vi "-Build_Query_Error.vi"(8 "error in (no error)":errorcluster, 11 "Postgres Connector In":refnum<class "Postgres Connector.lvclass">) -> (0 "error out":errorcluster, 3 "Postgres Connector Out":refnum<class "Postgres Connector.lvclass">)   [LabVIEW 2020, in "Postgres Connector.lvclass"]
doc: "This VI return the error associated with a query"
uses:
  Postgres Connector.lvclass
  Postgres Connector.lvclass/Postgres Connector.ctl
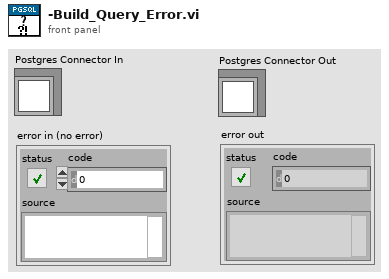
[diagram p1: front panel]
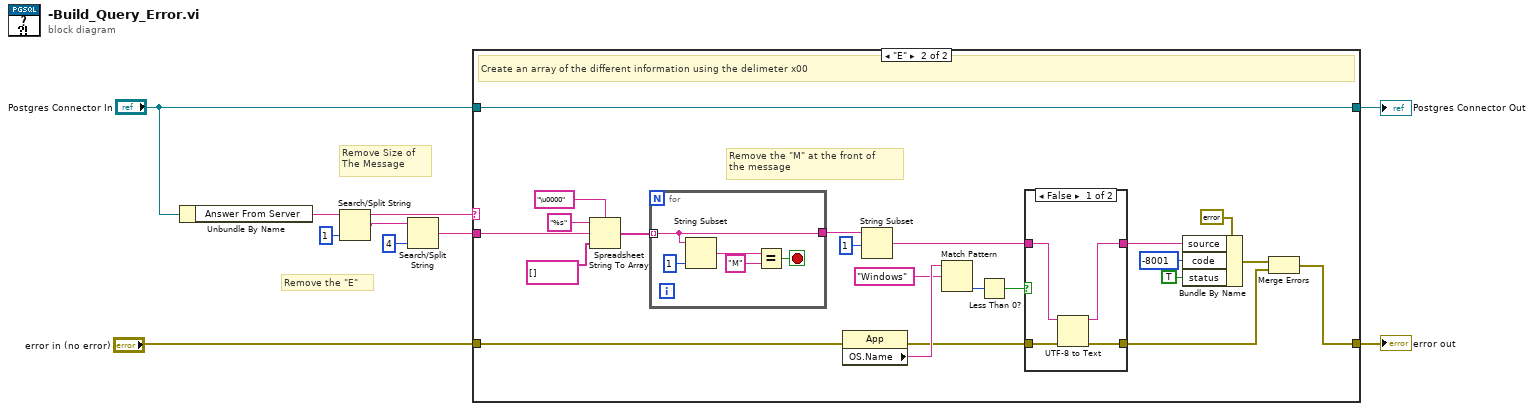
[diagram p0: block diagram]
diagram:
  # "Remove Size of\nThe Message"
  # "Remove the \"E\""
  n1 = Unbundle By Name("Postgres Connector In") -> ("Answer From Server"=w8:string)
  n2 = Search/Split String(string=w8, offset (0)=1 ("length (rest)")) -> (substring before match=w9:string, match + rest of string=w6:string)  [unwired: 1 in, 1 out]
  n3 = Search/Split String(string=w6, offset (0)=4 ("length (rest)")) -> (match + rest of string=w5:string)  [unwired: 1 in, 2 out]
  n4 = case shown="\"E\"" w9 {
    tunnel: "error in (no error)" -> [w12 w16]
    tunnel: [w12 w32] -> w4
    tunnel: w5 -> [_ w26]
    tunnel: "Postgres Connector In" -> [w11 w13]
    tunnel: [w11 w13] -> w1
    frame Default {
    }
    frame "E" {
      # "Remove the \"M\" at the front of\nthe message"
      # "Create an array of the different information using the delimeter x00"
      n5 = Spreadsheet String To Array(delimiter (Tab)="\u0000", format string="%s", spreadsheet string=w26, array type (2D Dbl)=string[] []) -> (array=w23:string[])
      n6 = for {
        tunnel: w23 -> [w43] mode=indexing
        tunnel: [w43] -> w24
        stop <- w41 stop-if-true
        n7 = String Subset(string=w43, length (rest)=1 ("length (rest)")) -> (substring=w44:string)  [unwired: 1 in]
        n8 = Equal?(x=w44, y="M") -> (x = y?=w41:bool)
      }
      n9 = property class="App"(error in=w16) -> (error out=w15:errorcluster, "OS.Name"=w18:string)  [unwired: 1 in, 1 out]
      n10 = String Subset(string=w24, offset (0)=1) -> (substring=w22:string)  [unwired: 1 in]
      n11 = Match Pattern(string=w18, regular expression="Windows") -> (offset past match=w19:i32)  [unwired: 1 in, 3 out]
      n12 = Less Than 0?(x=w19) -> (x < 0?=w20:bool)
      n13 = case shown="False" w20 {
        tunnel: [w38 w40] -> w21
        tunnel: w22 -> [w37 w40]
        tunnel: w15 -> [w36 w39]
        tunnel: [w35 w39] -> w14
        frame False {
          n14 = UTF-8 to Text(8:w36, 11:w37) -> (0:w35:errorcluster, 3:w38:string)  [unwired: 1 in]
        }
        frame True {
        }
      }
      n15 = Bundle By Name(cluster=errorcluster {"status"=FALSE, "code"=0, "source"=""} ("error in (no error)"), "source"=w21, "code"=-8001, "status"=TRUE) -> (w31:errorcluster)
      n16 = Merge Errors(w31, w14) -> (w32:errorcluster)
    }
  }
  "error out" <- w4
  "Postgres Connector Out" <- w1
